vi "SVT Swept Sine Engine (DAQmx).vi"(8 "error in (no error)":errorcluster, 9 "compute RMS levels (F)":bool, 11 "swept sine task in":T2={"source settings"={"AO task name"="", "source"=[]}, "stimulus settings"={"stimulus task name"="", "stimulus"=[]}, "response(s) settings"={"response task name"="", "response"=[]}, "measurement settings"={"AI sampling frequency"=51200.0, "AO sampling frequency"=51200.0, "AI block size"=10240, "AO block Size"=10240, "block duration [ms]"=200.0, "number of AI channels"=2, "device propagation delay [samples]"=0.0, "total propagation time [samples]"=0.0, "DUT propagation time [ms]"=0.0}, "linlog"=enum."linear", "repeat"=enum."off", "frequency list"=[800.0], "amplitude list"=[1.0], "settling time"={"settle time"=0.02, "settle cycles"=5}, "integration time"={"integration time"=0.02, "integration cycles"=5}, "frequencies indices"={"AI freq index"=0, "AO freq index"=0}, "read marks"={"write index"=51200, "read index"=20480, "freq start index"=20480, "freq stop index"=30720, "# extracted"=0, "buffer type"=enum."Invalid buffer", "read/write indices"=[{"settle time index"=29646, "integration time index"=30670}, {"settle time index"=0, "integration time index"=0}, {"settle time index"=0, "integration time index"=0}], "AO index"=1, "AI index"=0, "settled"=FALSE, "integration done"=FALSE}, "harmonic settings"={"maximum THD harmonic"=0, "harmonic mapping"=[], "units"={"THD unit"=enum."%", "nth harmonic unit"=enum."%", "SINAD unit"=enum."dB", "THD+N unit"=enum."dB"}}, "auto resolution settings"={"auto max step"=512, "slow threshold db"=6.0, "fast threshold db"=1.0}, "auto level settings"={"auto level enable"=FALSE, "auto level channel"=6, "ideal ref"=1.0, "max level"=10.0, "ref upper deviation db"=3.0, "ref lower deviation db"=-3.0}, "offset"=0.0, "ramping rate"=0.0, "phase"=0.0, "initialize"=FALSE} {"phase" format="%.2f"; "response(s) settings"."response"."channel info"."pregain" format="%.2f"; "response(s) settings"."response"."channel info"."weighting filter" items=["Linear", "A-weighting", "B-weighting", "C-weighting", "ITU-R 468-4", "Dolby", "CCITT", "C-message", "Wb", "Wc", "Wd", "We", "Wf", "Wh", "Wj", "Wk", "Wm", "AES17 20 kHz lowpass", "AES17 40 kHz lowpass", "AES17 20 kHz highpass", "AES17 40 kHz highpass"]; "response(s) settings"."response"."channel info"."dB reference" format="%^.1e"; "response(s) settings"."response"."channel info"."engineering units" items=["custom..."=0, "V"=1, "A"=21, "C"=30, "pC"=31, "s"=32, "-"=29, "Pa"=2, "N"=20, "g"=3, "m/s^2"=4, "m/s"=5, "m"=6, "mm/s"=12, "mm"=13, "micron/s"=14, "micron"=15, "in/s^2"=7, "in/s"=8, "in"=9, "mil/s"=10, "mil"=11, "rad/s^2"=16, "rad/s"=17, "rad"=18, "deg/s^2"=26, "deg/s"=27, "deg"=28, "RPM"=22, "cycle/s^2"=23, "Hz"=24, "cycle"=25, "strain"=19]; "response(s) settings"."response"."channel info"."sensor sensitivity" format="%#_5f"; "stimulus settings"."stimulus"."channel info"."pregain" format="%.2f"; "stimulus settings"."stimulus"."channel info"."weighting filter" items=["Linear", "A-weighting", "B-weighting", "C-weighting", "ITU-R 468-4", "Dolby", "CCITT", "C-message", "Wb", "Wc", "Wd", "We", "Wf", "Wh", "Wj", "Wk", "Wm", "AES17 20 kHz lowpass", "AES17 40 kHz lowpass", "AES17 20 kHz highpass", "AES17 40 kHz highpass"]; "stimulus settings"."stimulus"."channel info"."dB reference" format="%^.1e"; "stimulus settings"."stimulus"."channel info"."engineering units" items=["custom..."=0, "V"=1, "A"=21, "C"=30, "pC"=31, "s"=32, "-"=29, "Pa"=2, "N"=20, "g"=3, "m/s^2"=4, "m/s"=5, "m"=6, "mm/s"=12, "mm"=13, "micron/s"=14, "micron"=15, "in/s^2"=7, "in/s"=8, "in"=9, "mil/s"=10, "mil"=11, "rad/s^2"=16, "rad/s"=17, "rad"=18, "deg/s^2"=26, "deg/s"=27, "deg"=28, "RPM"=22, "cycle/s^2"=23, "Hz"=24, "cycle"=25, "strain"=19]; "stimulus settings"."stimulus"."channel info"."sensor sensitivity" format="%#_5f"; "ramping rate" format="%.4f"; "offset" format="%.2f"; "auto level settings"."ref lower deviation db" format="%.4f"; "auto level settings"."ref upper deviation db" format="%.4f"; "auto level settings"."max level" format="%.4f"; "auto level settings"."ideal ref" format="%.4f"; "auto resolution settings"."fast threshold db" format="%.4f"; "auto resolution settings"."slow threshold db" format="%.4f"; "harmonic settings"."maximum THD harmonic" max=10 step=1; "integration time"."integration time" format="%.2p"; "settling time"."settle time" format="%.2p"; "amplitude list" format="%.2f"; "frequency list" format="%.2f"; "measurement settings"."DUT propagation time [ms]" format="%.2f"; "measurement settings"."AO sampling frequency" format="%.2f"; "measurement settings"."AI sampling frequency" format="%.2f"}) -> (0 "error out":errorcluster, 1 "status":T1 {"% complete" format="%.2f"; "current processed frequency" format="%.2f"; "current source frequency" format="%.2f"; "elapsed time [s]" format="%.2f"}, 2 "swept sine measurements":T6 {"scaled response magnitude" format="%.3f"; "Harm[]" format="%.2f"; "THD" format="%.2f"; "Im [response]" format="%.2f"; "Re [response]" format="%.2f"; "Im [stimulus]" format="%.2f"; "Re [stimulus]" format="%.2f"; "RMS response" format="%.2f"; "RMS stimulus" format="%.2f"}, 3 "swept sine task out":T2={"source settings"={"AO task name"="", "source"=[]}, "stimulus settings"={"stimulus task name"="", "stimulus"=[]}, "response(s) settings"={"response task name"="", "response"=[]}, "measurement settings"={"AI sampling frequency"=51200.0, "AO sampling frequency"=51200.0, "AI block size"=10240, "AO block Size"=10240, "block duration [ms]"=200.0, "number of AI channels"=2, "device propagation delay [samples]"=0.0, "total propagation time [samples]"=0.0, "DUT propagation time [ms]"=0.0}, "linlog"=enum."linear", "repeat"=enum."off", "frequency list"=[800.0], "amplitude list"=[1.0], "settling time"={"settle time"=0.02, "settle cycles"=5}, "integration time"={"integration time"=0.02, "integration cycles"=5}, "frequencies indices"={"AI freq index"=0, "AO freq index"=0}, "read marks"={"write index"=61440, "read index"=30720, "freq start index"=30720, "freq stop index"=50176, "# extracted"=1024, "buffer type"=enum."Final buffer", "read/write indices"=[{"settle time index"=29646, "integration time index"=30670}, {"settle time index"=49102, "integration time index"=50126}, {"settle time index"=0, "integration time index"=0}], "AO index"=2, "AI index"=1, "settled"=TRUE, "integration done"=TRUE}, "harmonic settings"={"maximum THD harmonic"=0, "harmonic mapping"=[], "units"={"THD unit"=enum."%", "nth harmonic unit"=enum."%", "SINAD unit"=enum."dB", "THD+N unit"=enum."dB"}}, "auto resolution settings"={"auto max step"=512, "slow threshold db"=6.0, "fast threshold db"=1.0}, "auto level settings"={"auto level enable"=FALSE, "auto level channel"=6, "ideal ref"=1.0, "max level"=10.0, "ref upper deviation db"=3.0, "ref lower deviation db"=-3.0}, "offset"=0.0, "ramping rate"=0.0, "phase"=0.0, "initialize"=FALSE} {"phase" format="%.2f"; "response(s) settings"."response"."channel info"."pregain" format="%.2f"; "response(s) settings"."response"."channel info"."weighting filter" items=["Linear", "A-weighting", "B-weighting", "C-weighting", "ITU-R 468-4", "Dolby", "CCITT", "C-message", "Wb", "Wc", "Wd", "We", "Wf", "Wh", "Wj", "Wk", "Wm", "AES17 20 kHz lowpass", "AES17 40 kHz lowpass", "AES17 20 kHz highpass", "AES17 40 kHz highpass"]; "response(s) settings"."response"."channel info"."dB reference" format="%^.1e"; "response(s) settings"."response"."channel info"."engineering units" items=["custom..."=0, "V"=1, "A"=21, "C"=30, "pC"=31, "s"=32, "-"=29, "Pa"=2, "N"=20, "g"=3, "m/s^2"=4, "m/s"=5, "m"=6, "mm/s"=12, "mm"=13, "micron/s"=14, "micron"=15, "in/s^2"=7, "in/s"=8, "in"=9, "mil/s"=10, "mil"=11, "rad/s^2"=16, "rad/s"=17, "rad"=18, "deg/s^2"=26, "deg/s"=27, "deg"=28, "RPM"=22, "cycle/s^2"=23, "Hz"=24, "cycle"=25, "strain"=19]; "response(s) settings"."response"."channel info"."sensor sensitivity" format="%#_5f"; "stimulus settings"."stimulus"."channel info"."pregain" format="%.2f"; "stimulus settings"."stimulus"."channel info"."weighting filter" items=["Linear", "A-weighting", "B-weighting", "C-weighting", "ITU-R 468-4", "Dolby", "CCITT", "C-message", "Wb", "Wc", "Wd", "We", "Wf", "Wh", "Wj", "Wk", "Wm", "AES17 20 kHz lowpass", "AES17 40 kHz lowpass", "AES17 20 kHz highpass", "AES17 40 kHz highpass"]; "stimulus settings"."stimulus"."channel info"."dB reference" format="%^.1e"; "stimulus settings"."stimulus"."channel info"."engineering units" items=["custom..."=0, "V"=1, "A"=21, "C"=30, "pC"=31, "s"=32, "-"=29, "Pa"=2, "N"=20, "g"=3, "m/s^2"=4, "m/s"=5, "m"=6, "mm/s"=12, "mm"=13, "micron/s"=14, "micron"=15, "in/s^2"=7, "in/s"=8, "in"=9, "mil/s"=10, "mil"=11, "rad/s^2"=16, "rad/s"=17, "rad"=18, "deg/s^2"=26, "deg/s"=27, "deg"=28, "RPM"=22, "cycle/s^2"=23, "Hz"=24, "cycle"=25, "strain"=19]; "stimulus settings"."stimulus"."channel info"."sensor sensitivity" format="%#_5f"; "ramping rate" format="%.4f"; "offset" format="%.2f"; "auto level settings"."ref lower deviation db" format="%.4f"; "auto level settings"."ref upper deviation db" format="%.4f"; "auto level settings"."max level" format="%.4f"; "auto level settings"."ideal ref" format="%.4f"; "auto resolution settings"."fast threshold db" format="%.4f"; "auto resolution settings"."slow threshold db" format="%.4f"; "harmonic settings"."maximum THD harmonic" max=10 step=1; "integration time"."integration time" format="%.2p"; "settling time"."settle time" format="%.2p"; "amplitude list" format="%.2f"; "frequency list" format="%.2f"; "measurement settings"."DUT propagation time [ms]" format="%.2f"; "measurement settings"."AO sampling frequency" format="%.2f"; "measurement settings"."AI sampling frequency" format="%.2f"}, 4 "sweep done":bool, 5 "waveform data [V]":waveform(dbl)[](array[waveform]))   [LabVIEW 2017, in "SoundVib_SweptSine.lvlib"]
doc: "Performs swept-sine computations."
uses:
  <vilib>/addons/Sound and Vibration/svt_Swept Sine/SoundVib_SweptSine.lvlib
  <vilib>/addons/Sound and Vibration/svt_Swept Sine/subVIs/sv_Swept Sine Measurements.ctl
  <vilib>/addons/Sound and Vibration/svt_Swept Sine/subVIs/sv_Swept Sine Task.ctl
  <vilib>/addons/_NISVFA/_Shared subVIs/Controls/svc_Channel Info.ctl
  <vilib>/addons/_NISVFA/_Shared subVIs/Controls/svc_Engineering Units Text Ring.ctl
  <vilib>/addons/_NISVFA/_Shared subVIs/Controls/svc_Weighting Filter Text Ring.ctl
panel:
  in  "DBG (No DAQ)":bool
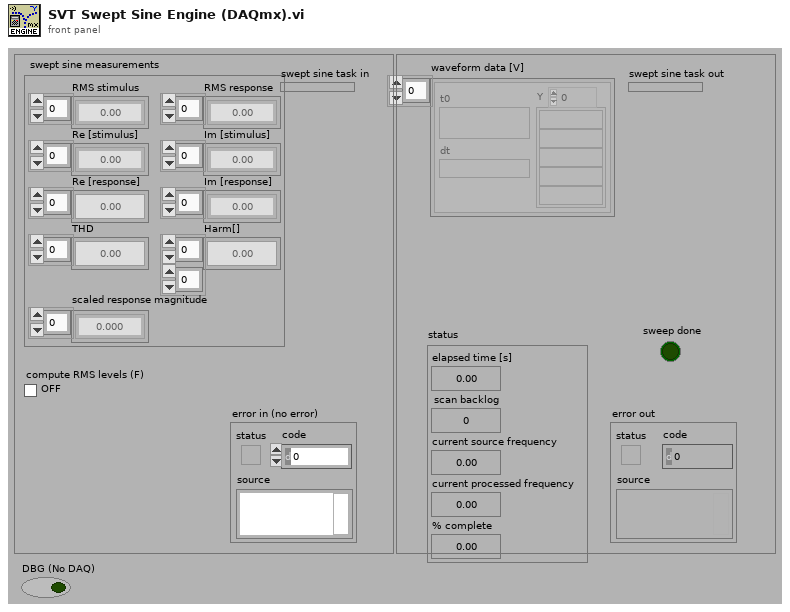
[diagram p1: front panel]
types:
  T1 = cluster{"elapsed time [s]":dbl, "scan backlog":u32, "current source frequency":dbl, "current processed frequency":dbl, "% complete":dbl}
  T2 = typedef "SoundVib_SweptSine.lvlib/sv_Swept Sine Task.ctl" = cluster{"source settings":cluster{"AO task name":refnum<k21>, "source":cluster{"AO physical channel":tag}[]}, "stimulus settings":cluster{"stimulus task name":refnum<k21>, "stimulus":cluster{"stimulus physical channel":tag, "channel info":T3}[]}, "response(s) settings":cluster{"response task name":refnum<k21>, "response":cluster{"response physical channel":tag, "channel info":T3}[]}, "measurement settings":cluster{"AI sampling frequency":dbl, "AO sampling frequency":dbl, "AI block size":i32, "AO block Size":i32, "block duration [ms]":dbl, "number of AI channels":i32, "device propagation delay [samples]":dbl, "total propagation time [samples]":dbl, "DUT propagation time [ms]":dbl}, "linlog":enum16{"linear", "log"}, "repeat":enum16{"off", "on"}, "frequency list":dbl[], "amplitude list":dbl[], "settling time":cluster{"settle time":dbl, "settle cycles":i32}, "integration time":cluster{"integration time":dbl, "integration cycles":i32}, "frequencies indices":cluster{"AI freq index":i32, "AO freq index":i32}, "read marks":cluster{"write index":u32, "read index":u32, "freq start index":u32, "freq stop index":u32, "# extracted":u32, "buffer type":enum16{"Invalid buffer", "Intermediate buffer", "Final buffer"}, "read/write indices":cluster{"settle time index":u32, "integration time index":u32}[], "AO index":i32, "AI index":i32, "settled":bool, "integration done":bool}, "harmonic settings":cluster{"maximum THD harmonic":u32, "harmonic mapping":u32[], "units":cluster{"THD unit":enum16{"dB", "%"}, "nth harmonic unit":enum16{"dB", "%"}, "SINAD unit":enum16{"dB", "%"}, "THD+N unit":enum16{"dB", "%"}}}, "auto resolution settings":cluster{"auto max step":i32, "slow threshold db":dbl, "fast threshold db":dbl}, "auto level settings":cluster{"auto level enable":bool, "auto level channel":u8, "ideal ref":sgl, "max level":sgl, "ref upper deviation db":sgl, "ref lower deviation db":sgl}, "offset":dbl, "ramping rate":dbl, "phase":dbl, "initialize":bool}
  T3 = typedef "svc_Channel Info.ctl" = cluster{"sensor sensitivity":dbl, "engineering units":T4, "dB reference":dbl, "custom label":string, "weighting filter":T5, "pregain":dbl}
  T4 = typedef "svc_Engineering Units Text Ring.ctl" = u16
  T5 = typedef "svc_Weighting Filter Text Ring.ctl" = u16
  T6 = typedef "SoundVib_SweptSine.lvlib/sv_Swept Sine Measurements.ctl" = cluster{"RMS stimulus":dbl[], "RMS response":dbl[], "Re [stimulus]":dbl[], "Im [stimulus]":dbl[], "Re [response]":dbl[], "Im [response]":dbl[], "THD":dbl[], "Harm[]":dbl[][], "scaled response magnitude":dbl[]}
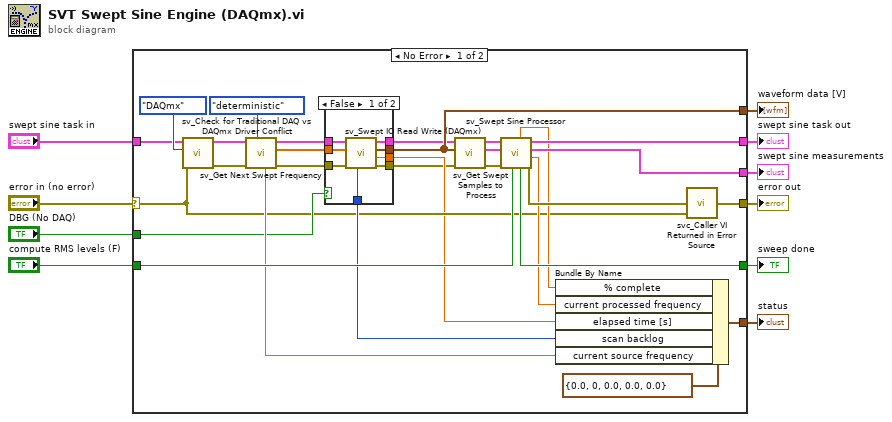
[diagram p0: block diagram]
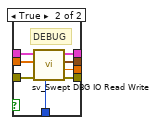
[diagram p2: hidden frame]
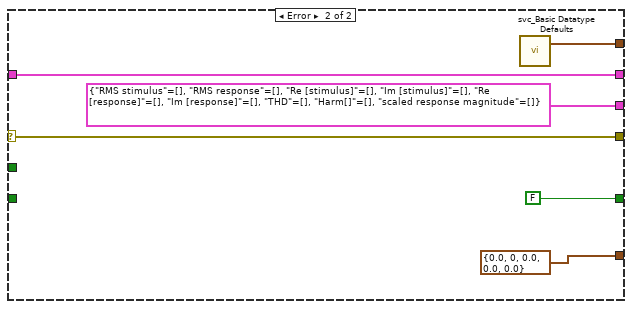
[diagram p3: hidden frame]
diagram:
  n1 = case shown="No Error" "error in (no error)" {
    selector: "error in (no error)" -> [w14 w59]
    tunnel: "compute RMS levels (F)" -> [w39 _]
    tunnel: [w38 w61] -> w9
    tunnel: [w37 FALSE ("sweep done")] -> w8
    tunnel: "swept sine task in" -> [w17 w61]
    tunnel: [w31 T1 {"elapsed time [s]"=0.0, "scan backlog"=0, "current source frequency"=0.0, "current processed frequency"=0.0, "% complete"=0.0} ("status")] -> w6
    tunnel: [w30 T6 {"RMS stimulus"=[], "RMS response"=[], "Re [stimulus]"=[], "Im [stimulus]"=[], "Re [response]"=[], "Im [response]"=[], "THD"=[], "Harm[]"=[], "scaled response magnitude"=[]} ("swept sine measurements")] -> w5
    tunnel: [w28 w59] -> w4
    tunnel: [w25 w56] -> w3
    tunnel: "DBG (No DAQ)" -> [w23 _]
    frame No Error {
      n2 = call <vilib>:"sv_Check for Traditional DAQ vs DAQmx Driver Conflict.vi"("error in (no error)"=w14, "device driver"=enum16{"DAQmx", "Traditional DAQ"}."DAQmx", "swept sine task"=w17) -> ("error out"=w15:errorcluster, "dup swept sine task"=w16:T2)  [unwired: 7 in]
      n3 = call <vilib>:"sv_Get Next Swept Frequency.vi"("mode"=enum16{"feedback", "deterministic"}."deterministic", "error in (no error)"=w15, "swept sine task in"=w16) -> ("error out"=w27:errorcluster, "stimulus"=w11:dbl[], "swept sine task out"=w26:T2, "current source frequency"=w33:dbl)  [unwired: 5 in]
      n4 = case shown="False" w23 {
        tunnel: w27 -> [w46 w53]
        tunnel: [w45 w50] -> w12
        tunnel: w26 -> [w47 w55]
        tunnel: [w44 w52] -> w22
        tunnel: [w43 w48] -> w25
        tunnel: [w42 w51] -> w13
        tunnel: [w41 w49] -> w24
        tunnel: w11 -> [w40 w54]
        frame False {
          n5 = call <vilib>:"sv_Swept IO Read Write (DAQmx).vi"("error in (no error)"=w46, "stimulus"=w40, "swept sine task in"=w47) -> ("error out"=w45:errorcluster, "elapsed time"=w42:dbl, "waveform data [V]"=w43:waveform(dbl)[], "swept sine task out"=w44:T2, "scan backlog"=w41:u32)  [unwired: 4 in]
        }
        frame True {
          # "DEBUG"
          n6 = call <vilib>:"sv_Swept DBG IO Read Write.vi"("error in (no error)"=w53, "stimulus"=w54, "swept sine task in"=w55) -> ("error out"=w50:errorcluster, "elapsed time"=w51:dbl, "waveform data [V]"=w48:waveform(dbl)[], "swept sine task out"=w52:T2, "scan backlog"=w49:u32)  [unwired: 4 in]
        }
      }
      n7 = call <vilib>:"sv_Get Swept Samples to Process.vi"("error in (no error)"=w12, "waveform data [V]"=w25, "swept sine task in"=w22) -> ("error out"=w36:errorcluster, "data to process [V]"=w34:cluster{"stimulus":dbl[], "response":dbl[]}, "swept sine task out"=w35:T2)  [unwired: 6 in]
      n8 = call <vilib>:"sv_Swept Sine Processor.vi"("RMS level"=w39, "error in (no error)"=w36, "data to process [V]"=w34, "swept sine task in"=w35) -> ("error out"=w29:errorcluster, "processed frequency (Hz)"=w20:dbl, "swept sine measurements"=w30:T6, "swept sine task out"=w38:T2, "sweep done"=w37:bool, "%done"=w21:dbl)  [unwired: 2 in]
      n9 = Bundle By Name(cluster=T1 {"elapsed time [s]"=0.0, "scan backlog"=0, "current source frequency"=0.0, "current processed frequency"=0.0, "% complete"=0.0} ("status"), "% complete"=w21, "current processed frequency"=w20, "elapsed time [s]"=w13, "scan backlog"=w24, "current source frequency"=w33) -> (w31:T1)
      n10 = call <vilib>:"svc_Caller VI Returned in Error Source.vi"("warning input to caller"=w14, "error in (no error)"=w29) -> ("error out"=w28:errorcluster)  [unwired: 3 in]
    }
    frame Error {
      n11 = call <vilib>:"svc_Basic Datatype Defaults.vi"() -> ("empty array of waveforms"=w56:waveform(dbl)[])  [unwired: 7 in, 12 out]
    }
  }
  "swept sine measurements" <- w5
  "swept sine task out" <- w9
  "error out" <- w4
  "sweep done" <- w8
  "waveform data [V]" <- w3
  "status" <- w6
